vi "Read Left Joystick Axis.vi"(8 "error in (no error)":errorcluster, 11 "XboxController-V in":refnum<class "XboxController-V.lvclass">) -> (0 "error out":errorcluster, 2 "Joystick Axis":T1 {"Y" scale=-1.0..1.0; "X" scale=-1.0..1.0}, 3 "XboxController-V out":refnum<class "XboxController-V.lvclass">)   [LabVIEW 2013, in "XboxController-V.lvclass"]
uses:
  XboxController-V.lvclass
  Logical Systems/XBoxController/JoystickAxis.ctl
  XboxController-V.lvclass/XboxController-V.ctl
  Logical Systems/XBoxController/XBoxController.lvclass
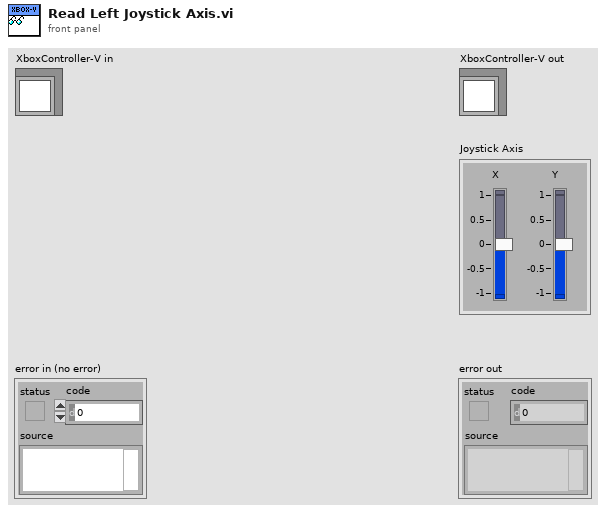
[diagram p1: front panel]
types:
  T1 = typedef "XBoxController.lvclass/JoystickAxis.ctl" = cluster{"X":dbl, "Y":dbl}
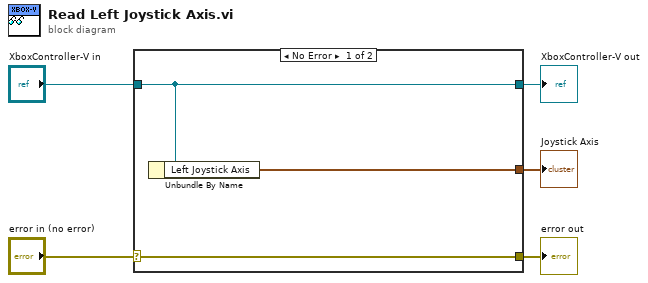
[diagram p0: block diagram]
diagram:
  n1 = case shown="No Error" "error in (no error)" {
    selector: "error in (no error)" -> [w8 w9]
    tunnel: [w8 w9] -> w4
    tunnel: [w7 w10] -> w2
    tunnel: "XboxController-V in" -> [w7 w10]
    tunnel: [w6 _] -> w1
    frame No Error {
      n2 = Unbundle By Name(w7) -> ("Left Joystick Axis"=w6:T1)
    }
    frame Error {
    }
  }
  "error out" <- w4
  "XboxController-V out" <- w2
  "Joystick Axis" <- w1
